vi "init.vi"(8 "error in (no error)":errorcluster, 11 "MsgUserEventStopMechanism In":refnum<class "MsgUserEventStopMechanism.lvclass">) -> (0 "error out":errorcluster, 3 "MsgUserEventStopMechanism Out":refnum<class "MsgUserEventStopMechanism.lvclass">)   [LabVIEW 2023, in "TLC_Daemon.lvlib" / "MsgUserEventStopMechanism.lvclass"]
doc: "Initializes the stop mechanism.\n_____________________________________\nTLC Daemon 1.0.0.2\nCopyright (c) 2026 Andrea Cadei"
uses:
  MsgUserEventStopMechanism.lvclass
  MsgUserEventStopMechanism.lvclass/MsgUserEventStopMechanism.ctl
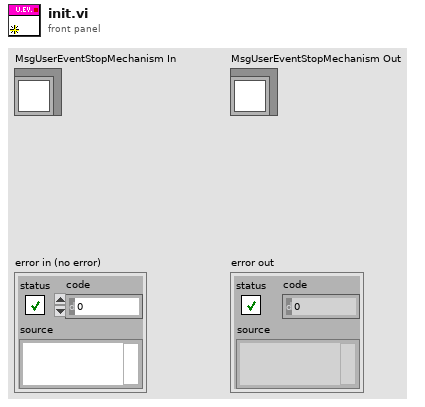
[diagram p1: front panel]
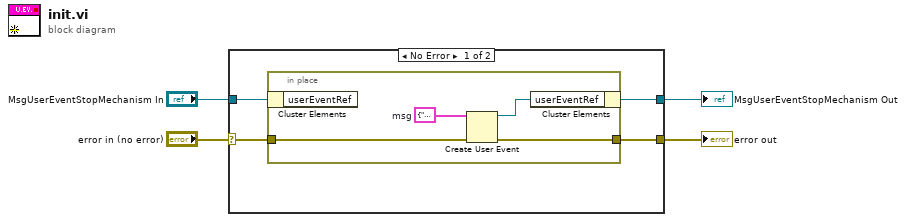
[diagram p0: block diagram]
diagram:
  n1 = case shown="No Error" "error in (no error)" {
    selector: "error in (no error)" -> [w5 w14]
    tunnel: [w8 w14] -> w4
    tunnel: [w7 w13] -> w1
    tunnel: "MsgUserEventStopMechanism In" -> [w6 w13]
    frame No Error {
      n2 = in-place {
        in-place-border: w5 -> [w12]
        in-place-border: [w11] -> w8
        w9 = cluster{"message":string, "data":variant} {"message"="", "data"=variant}  # msg
        n3 = in-place-cluster #1(w6) -> ()  [unwired: 1 out]
        n4 = Create User Event(user event datatype=w9, error in=w12) -> (user event=w10:refnum<user-event>, error out=w11:errorcluster)
        n5 = in-place-cluster #1("userEventRef"=w10) -> (w7:refnum<class "MsgUserEventStopMechanism.lvclass">)
      }
    }
    frame Error {
    }
  }
  "error out" <- w4
  "MsgUserEventStopMechanism Out" <- w1
